vi "Configure Single Assert Display.vi"(8 "error in (no error)":errorcluster, 10 "Assert UID":string) -> (0 "error out":errorcluster, 3 "Single Assert Display out":refnum<class "Single Assert Display.lvclass">)   [LabVIEW 2016, in "Assert API Components.lvlib" / "Assert Display.lvlib" / "Single Assert Display.lvlib" / "Single Assert Display.lvclass"]
uses:
  Single Assert Display.lvclass
  Single Assert Display.lvclass/Single Assert Display.ctl
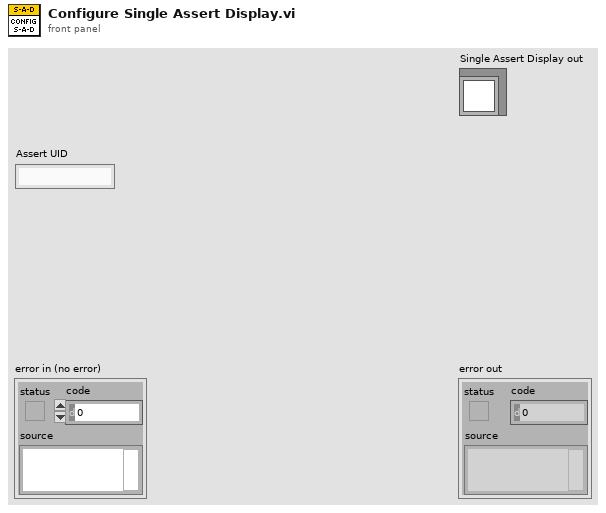
[diagram p1: front panel]
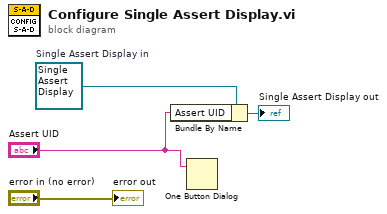
[diagram p0: block diagram]
diagram:
  w3 = refnum<class "Single Assert Display.lvclass"> refnum  # Single Assert Display in
  n1 = Bundle By Name(cluster=w3, "Assert UID"="Assert UID") -> (→"Single Assert Display out":refnum<class "Single Assert Display.lvclass">)
  n2 = One Button Dialog(message="Assert UID") -> ()  [unwired: 1 in, 1 out]
  "error out" <- "error in (no error)"
